vi "RS_SMBV100A_CalculateAcrScenario.vi"(8 "Start speed":dbl=10.0, 9 "Z":dbl, 10 "Y":dbl=10.0, 11 "X":dbl=10.0) -> (3 "Duration":dbl)   [LabVIEW 2018]
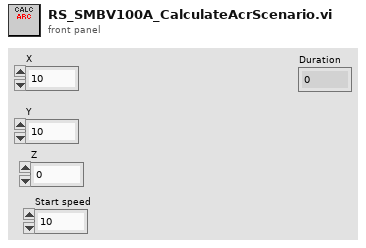
[diagram p1: front panel]
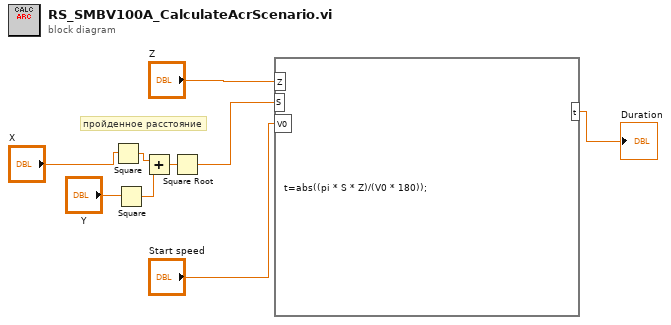
[diagram p0: block diagram]
diagram:
  # "пройденное расстояние"
  n1 = Square(x="X") -> (x^2=w8:dbl)
  n2 = Square(x="Y") -> (x^2=w7:dbl)
  n3 = Add(x=w8, y=w7) -> (x+y=w9:dbl)
  n4 = Square Root(x=w9) -> (sqrt(x)=w3:dbl)
  n5 = formula code="t=abs((pi * S * Z)/(V0 * 180));"("Z"="Z", "S"=w3, "V0"="Start speed") -> ("t"=→"Duration":dbl)
